vi "Read Transform.vi"(8 "error in (no error)":errorcluster, 11 "SimulationObject in":refnum<class "SimulationObject.lvclass">) -> (0 "error out":errorcluster, 2 "Transform out":refnum<class "Transform.lvclass">, 3 "SimulationObject out":refnum<class "SimulationObject.lvclass">)   [LabVIEW 2022 SP3, in "SimulationObject.lvclass"]
uses:
  SimulationObject.lvclass
  Components/Transform/Transform.lvclass
  SimulationObject.lvclass/SimulationObject.ctl
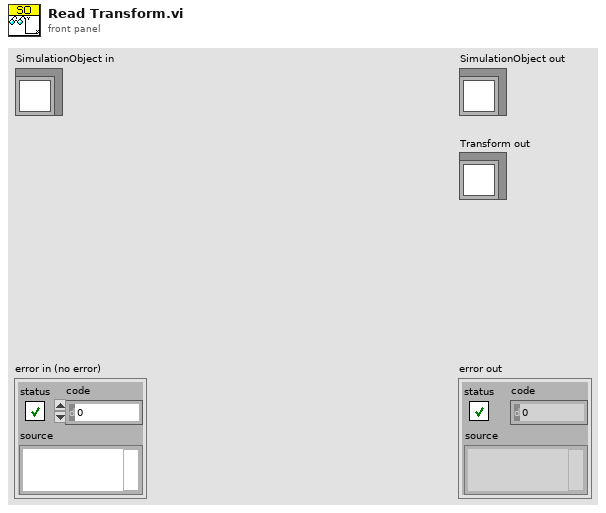
[diagram p1: front panel]
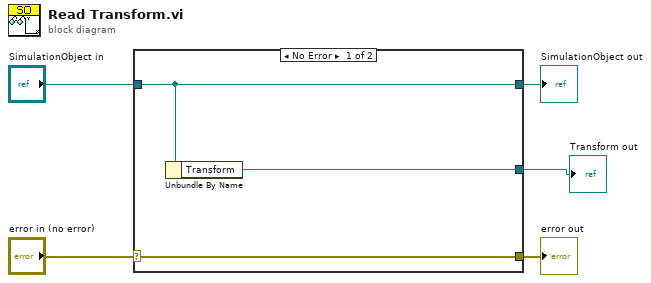
[diagram p0: block diagram]
diagram:
  n1 = case shown="No Error" "error in (no error)" {
    selector: "error in (no error)" -> [w8 w9]
    tunnel: [w8 w9] -> w4
    tunnel: [w7 w10] -> w2
    tunnel: "SimulationObject in" -> [w7 w10]
    tunnel: [w6 _] -> w1
    frame No Error {
      n2 = Unbundle By Name(w7) -> ("Transform"=w6:refnum<class "Transform.lvclass">)
    }
    frame Error {
    }
  }
  "error out" <- w4
  "SimulationObject out" <- w2
  "Transform out" <- w1
